vi "RFIDSetAntennaEnabled.vi"(0 "error in (no error)":errorcluster, 2 "AntennaState":bool caption="Antenna Enabled", 3 "Device In":u64) -> (7 "error out":errorcluster, 10 "Device Out":u64)   [LabVIEW 2012, in "Phidget RFID.lvlib"]
doc: "${AntennaEnabled:Header}"
uses:
  <instrlib>/Phidgets/Phidget RFID/Phidget RFID.lvlib
  <instrlib>/Phidgets/Phidget Common/Phidget Common.lvlib
  phidget22.dll
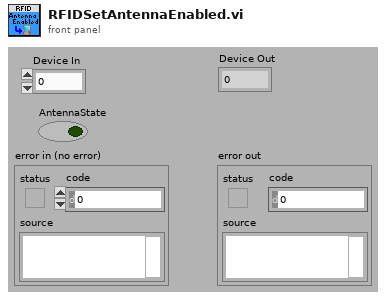
[diagram p1: front panel]
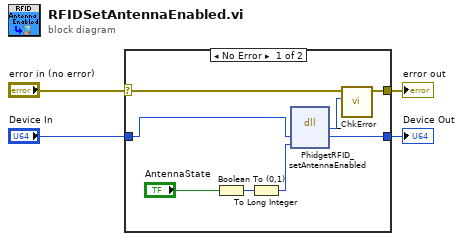
[diagram p0: block diagram]
diagram:
  n1 = case shown="No Error" "error in (no error)" {
    selector: "error in (no error)" -> [w9 w14]
    tunnel: [w8 w14] -> w3
    tunnel: "Device In" -> [w12 w13]
    tunnel: [w11 w13] -> w1
    frame No Error {
      n2 = Boolean To (0,1)(Boolean="AntennaState") -> (0, 1=w7:i16)
      n3 = To Long Integer(number=w7) -> (32bit integer=w6:i32)
      n4 = dll-call lib="phidget22.*" fn="PhidgetRFID_setAntennaEnabled"("phid"=w12, "setEngaged"=w6) -> ("return type"=w10:i32, "phid"=w11:u64)  [unwired: 4 in, 2 out]
      n5 = call <instrlib>:"_ChkError.vi"("Return Code"=w10, "error in (no error)"=w9) -> ("error out"=w8:errorcluster)  [unwired: 9 in]
    }
    frame Error {
    }
  }
  "error out" <- w3
  "Device Out" <- w1
